vi "Main.vi"() -> ()   [LabVIEW 2022 SP3]
uses:
  MsgTypedef.ctl
  ProcessDataTypedef.ctl
  <vilib>/MakerHub/LINX/Private/Type Defs/LINX Ref.ctl
  <vilib>/MakerHub/LINX/Private/Type Defs/Platform.ctl
  <vilib>/MakerHub/LINX/Private/Type Defs/Interface.ctl
  <vilib>/MakerHub/LINX/Private/Device/Type Defs/LINX Device Config.ctl
  <vilib>/MakerHub/LINX/Private/Device/Type Defs/TCP Config.ctl
  <vilib>/MakerHub/LINX/Private/Device/Type Defs/Channels.ctl
  <vilib>/MakerHub/LINX/Public/Peripherals/Analog/Analog Read 1 Chan.vi
  <vilib>/MakerHub/LINX/Public/Peripherals/Digital/Digital Read 1 Chan.vi
  <vilib>/MakerHub/LINX/Public/Peripherals/Digital/Digital Write 1 Chan.vi
  <vilib>/MakerHub/LINX/Public/Peripherals/Analog/Analog Read N Chans.vi
  <vilib>/MakerHub/LINX/Public/Peripherals/Digital/Digital Read N Chans.vi
  <vilib>/MakerHub/LINX/Public/Peripherals/Digital/Digital Write N Chans.vi
  <vilib>/MakerHub/LINX/Private/Local IO/LinxAnalogRead.vi
  <vilib>/MakerHub/LINX/Public/Utilities/Check Channel.vi
  <vilib>/MakerHub/LINX/Private/Local IO/LinxDigitalRead.vi
  <vilib>/MakerHub/LINX/Private/Local IO/LinxDigitalWrite.vi
  <vilib>/MakerHub/LINX/Public/Utilities/Open Serial.vi
  <vilib>/MakerHub/LINX/Private/Utilties/Generate Error.vi
  <vilib>/MakerHub/LINX/LMH-LINX.lvlib
  <vilib>/MakerHub/LINX/Private/Device/Device.lvlib
panel:
  out "Loop Rate (Hz)":u32
  in  "Close":bool
  in  "Link":bool
  in  "AI Channel":u8
  out "Analog Data":dbl(graph)
  in  "DI Channel":u8=2
  out "DI Value":bool
  in  "DO Value":bool
  in  "DO Channel":u8=13
  in  "Serial Port":refnum<visa-resource-name>
  # "需求....\n1. linx 連結Arduino board \n2. 即時反應IO狀態\n3. 從VI panel 下達IO控制\n4. 可能作狀態觸發 record 記錄到檔案？\n5. 其它想法...."
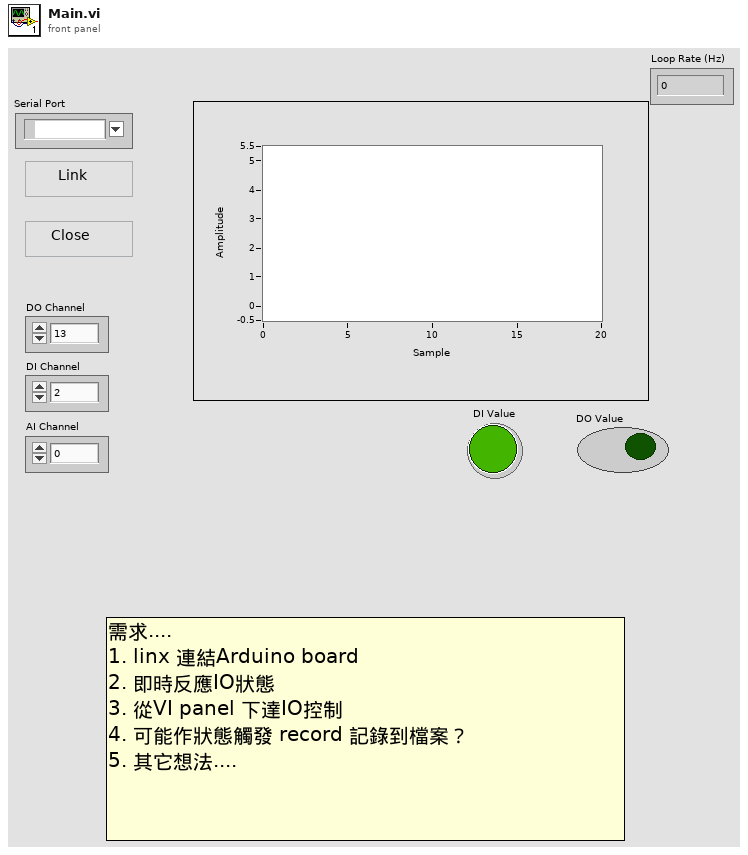
[diagram p1: front panel]
types:
  T1 = typedef "MsgTypedef.ctl" = cluster{"CMD":string, "DATA":variant}
  T2 = typedef "ProcessDataTypedef.ctl" = cluster{"SerialPort":refnum<visa-resource-name>, "DO Channel":u8, "DI Channel":u8, "AI Channel":u8, "AIValue":dbl, "DOStatus":bool, "DIStatus":bool, "DeviceName":string, "LINXResource":T3}
  T3 = typedef "LMH-LINX.lvlib/LINX Ref.ctl" = cluster{"IO":T4, "Interface":T5, "LINX Device Config":T6}
  T4 = typedef "LMH-LINX.lvlib/Platform.ctl" = enum16{"Remote", "Local"}
  T5 = typedef "LMH-LINX.lvlib/Interface.ctl" = enum16{"Serial", "TCP"}
  T6 = typedef "LMH-LINX.lvlib/Device.lvlib/LINX Device Config.ctl" = cluster{"Interface":T5, "COM Port":refnum<visa-resource-name>, "TCP Configuration":T7, "Device Family":u8, "Device ID":u8, "Device Name":string, "TCP Ref":refnum<k5>, "Channels":T8}
  T7 = typedef "LMH-LINX.lvlib/Device.lvlib/TCP Config.ctl" = cluster{"IP Address":string, "Port":u16}
  T8 = typedef "LMH-LINX.lvlib/Channels.ctl" = cluster{"DI":u8[], "DO":u8[], "AI":u8[], "AO":u8[], "PWM":u8[], "QE":u8[], "UART":u8[], "I2C 2":u8[], "SPI":u8[], "CAN":u8[], "Servo":u8[], "AI Ref (V)":dbl, "AI Resolution (Bits)":u8, "AO Ref (V)":dbl, "AO Resolution (Bits)":u8}
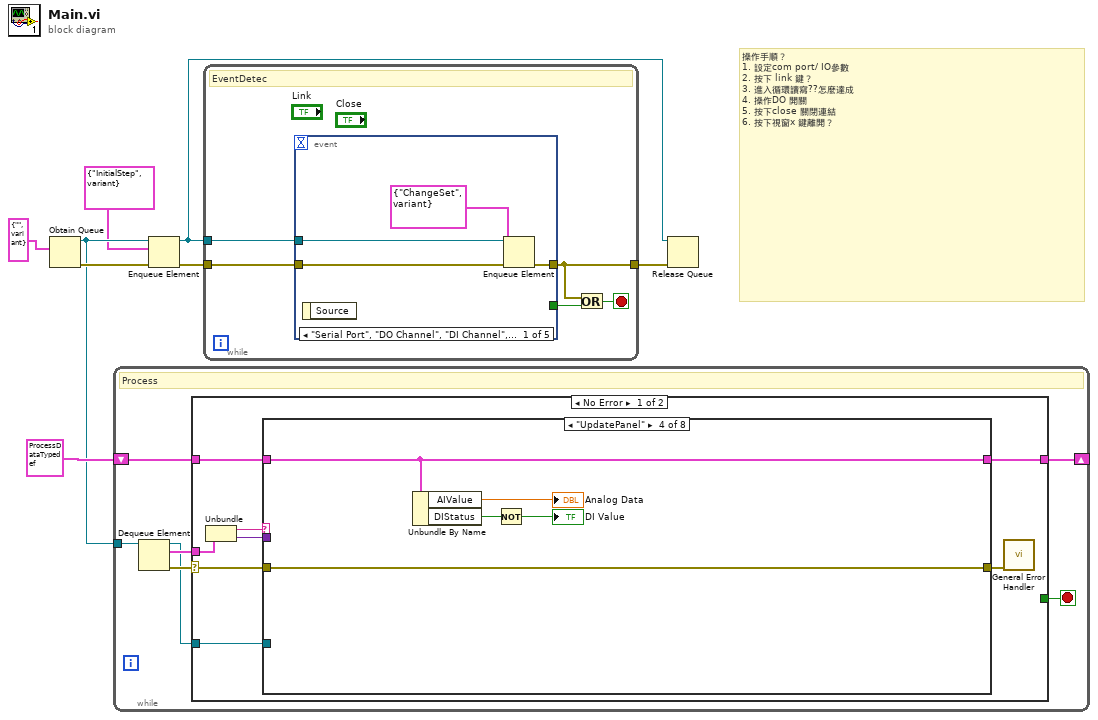
[diagram p0: block diagram]
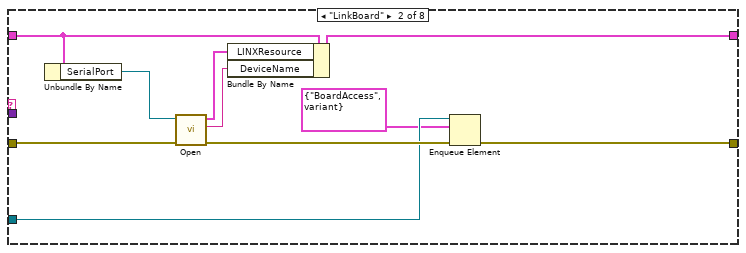
[diagram p3: hidden frame]
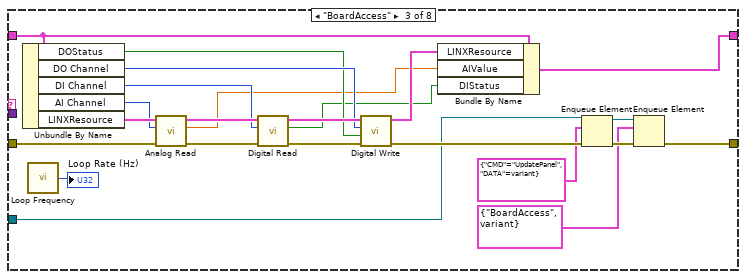
[diagram p4: hidden frame]
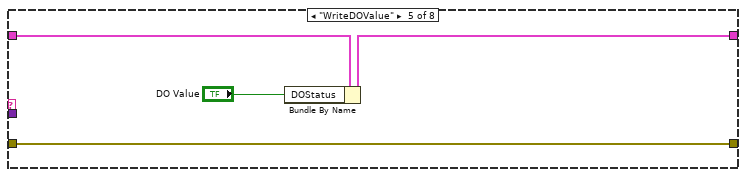
[diagram p5: hidden frame]
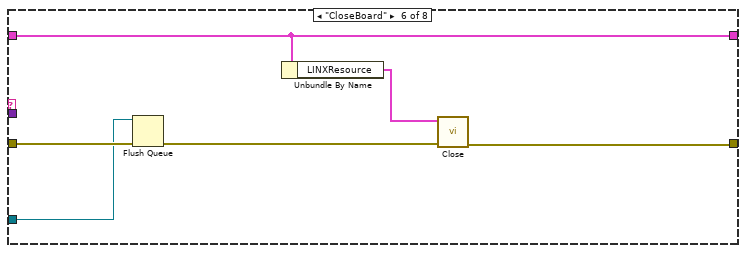
[diagram p6: hidden frame]
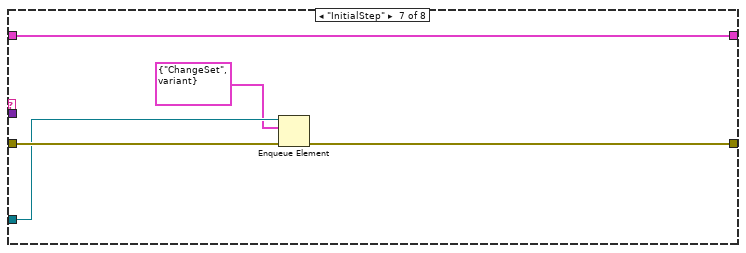
[diagram p7: hidden frame]
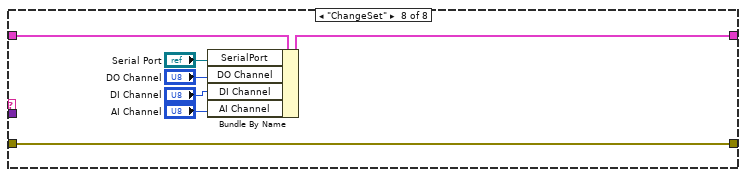
[diagram p8: hidden frame]
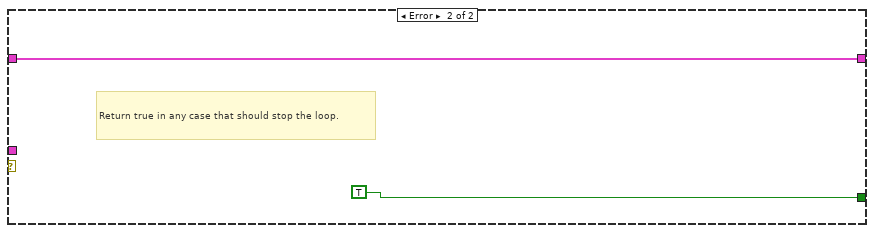
[diagram p9: hidden frame]
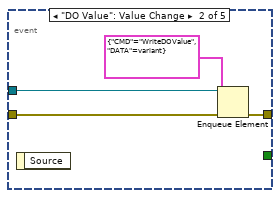
[diagram p10: hidden frame]
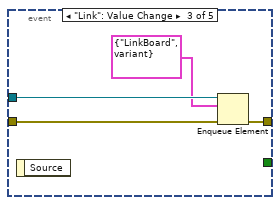
[diagram p11: hidden frame]
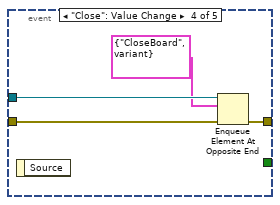
[diagram p12: hidden frame]
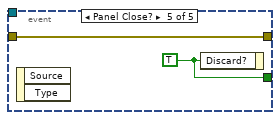
[diagram p13: hidden frame]
diagram:
  # "操作手順？\n1. 設定com port/ IO參數\n2. 按下 link 鍵？\n3. 進入循環讀寫??怎麼達成\n4. 操作DO 開關\n5. 按下close 關閉連結\n6. 按下視窗x 鍵離開？"
  n1 = Obtain Queue(element data type=T1 {"CMD"="", "DATA"=variant}) -> (queue out=w2:refnum<queue>, error out=w8:errorcluster)  [unwired: 4 in, 1 out]
  n2 = while {
    tunnel: w2 -> [w15]
    shift-right: [w11] -> _
    shift-left: T2 {"SerialPort"="", "DO Channel"=13, "DI Channel"=2, "AI Channel"=0, "AIValue"=0.0, "DOStatus"=FALSE, "DIStatus"=FALSE, "DeviceName"="", "LINXResource"={"IO"=enum."Remote", "Interface"=enum."Serial", "LINX Device Config"={"Interface"=enum."Serial", "COM Port"="COM13", "TCP Configuration"={"IP Address"="", "Port"=0}, "Device Family"=1, "Device ID"=1, "Device Name"="myRIO-1900", "TCP Ref"=refnum, "Channels"={"DI"=[0, 1, 2, 3, 4, 5, 6, 7, 8, 9, 10, 11, 12, 13, 14, 15, 16, 17, 18, 19, 20, 21, 22, 23, 24, 25, 26, 27, 28, 29, 30, 31, 32, 33, 34, 35, 36, 37, 38, 39, 40, 41, 42, 43, 44, 45, 46], "DO"=[0, 1, 2, 3, 4, 5, 6, 7, 8, 9, 10, 11, 12, 13, 14, 15, 16, 17, 18, 19, 20, 21, 22, 23, 24, 25, 26, 27, 28, 29, 30, 31, 32, 33, 34, 35, 36, 37, 38, 39, 40, 41, 42, 43, 44, 45, 46], "AI"=[0, 1, 2, 3, 4, 5, 6, 7, 8, 9, 10, 11], "AO"=[], "PWM"=[3, 5, 6, 9, 10], "QE"=[], "UART"=[0, 1], "I2C 2"=[0], "SPI"=[0], "CAN"=[], "Servo"=[], "AI Ref (V)"=0.0, "AI Resolution (Bits)"=0, "AO Ref (V)"=0.0, "AO Resolution (Bits)"=0}}}} -> [w10]
    stop <- w12 stop-if-true
    # "Process"
    n3 = Dequeue Element(queue=w15) -> (queue out=w9:refnum<queue>, element=w13:T1, error out=w14:errorcluster)  [unwired: 2 in, 1 out]
    n4 = case shown="No Error" w14 {
      selector: w14 -> [w21 _]
      tunnel: w13 -> [w23 _]
      tunnel: [_ TRUE] -> w12
      tunnel: [w20 w86] -> w11
      tunnel: w10 -> [w19 w86]
      tunnel: w9 -> [w17 _]
      frame No Error {
        n5 = Unbundle(w23) -> ("CMD"=w22:string, "DATA"=w18:variant)
        n6 = case shown="\"UpdatePanel\"" w22 {
          tunnel: w21 -> [w24 w35 w53 w63 w66 w73 w77 w79]
          tunnel: [w25 w31 w50 w62 w65 w71 w78 w84] -> w20
          tunnel: w19 -> [w25 w33 w52 w62 w67 w71 w78 w85]
          tunnel: w18 -> [_ _ _ _ _ _ _ _]
          tunnel: [w24 w28 w38 w63 w66 w72 w76 w79] -> w16
          tunnel: w17 -> [_ w27 w40 _ _ w68 w75 _]
          frame Default {
          }
          frame "LinkBoard" {
            n7 = Unbundle By Name(w33) -> ("SerialPort"=w32:refnum<visa-resource-name>)
            n8 = call-poly <vilib>:"Open.vi"("Error In"=w35, "Serial Port"=w32) -> ("Error Out"=w34:errorcluster, "Device Name"=w29:string, "LINX Resource"=w30:T3)  [unwired: 7 in]
            n9 = Bundle By Name(cluster=w33, "LINXResource"=w30, "DeviceName"=w29) -> (w31:T2)
            n10 = Enqueue Element(queue=w27, element=T1 {"CMD"="BoardAccess", "DATA"=variant}, error in (no error)=w34) -> (error out=w28:errorcluster)  [unwired: 1 in, 2 out]
          }
          frame "BoardAccess" {
            n11 = Unbundle By Name(w52) -> ("DOStatus"=w45:bool, "DO Channel"=w46:u8, "DI Channel"=w47:u8, "AI Channel"=w48:u8, "LINXResource"=w51:T3)
            n12 = call <vilib>:"Loop Frequency.vi"() -> ("Loop Rate (Hz)"=→"Loop Rate (Hz)":u32)
            n13 = call-poly <vilib>:"Analog Read.vi"("Error In"=w53, "Analog Channel"=w48, "LINX Resource"=w51) -> ("Error Out"=w57:errorcluster, "Voltage"=w44:dbl, "LINX Resource"=w58:T3)  [unwired: 5 in, 1 out]
            n14 = call-poly <vilib>:"Digital Read.vi"("Error In"=w57, "DI Channel"=w47, "LINX Resource"=w58) -> ("Error Out"=w55:errorcluster, "DI Value"=w43:bool, "LINX Resource"=w56:T3)  [unwired: 6 in]
            n15 = call-poly <vilib>:"Digital Write.vi"("Error In"=w55, "Output Value"=w45, "DO Channel"=w46, "LINX Resource"=w56) -> ("Error Out"=w54:errorcluster, "LINX Resource"=w49:T3)  [unwired: 6 in]
            n16 = Bundle By Name(cluster=w52, "LINXResource"=w49, "AIValue"=w44, "DIStatus"=w43) -> (w50:T2)
            n17 = Enqueue Element(queue=w40, element=T1 {"CMD"="UpdatePanel", "DATA"=variant}, error in (no error)=w54) -> (queue out=w37:refnum<queue>, error out=w41:errorcluster)  [unwired: 1 in, 1 out]
            n18 = Enqueue Element(queue=w37, element=T1 {"CMD"="BoardAccess", "DATA"=variant}, error in (no error)=w41) -> (error out=w38:errorcluster)  [unwired: 1 in, 2 out]
          }
          frame "UpdatePanel" {
            n19 = Unbundle By Name(w62) -> ("AIValue"=→"Analog Data":dbl, "DIStatus"=w61:bool)
            n20 = Not(x=w61) -> (.not. x?=→"DI Value":bool)
          }
          frame "WriteDOValue" {
            n21 = Bundle By Name(cluster=w67, "DOStatus"="DO Value") -> (w65:T2)
          }
          frame "CloseBoard" {
            n22 = Flush Queue(queue=w68, error in (no error)=w73) -> (error out=w69:errorcluster)  [unwired: 2 out]
            n23 = Unbundle By Name(w71) -> ("LINXResource"=w70:T3)
            n24 = call <vilib>:"Close.vi"("Error In"=w69, "LINX Resource"=w70) -> ("Error Out"=w72:errorcluster)  [unwired: 9 in]
          }
          frame "InitialStep" {
            n25 = Enqueue Element(queue=w75, element=T1 {"CMD"="ChangeSet", "DATA"=variant}, error in (no error)=w77) -> (error out=w76:errorcluster)  [unwired: 1 in, 2 out]
          }
          frame "ChangeSet" {
            n26 = Bundle By Name(cluster=w85, "SerialPort"="Serial Port", "DO Channel"="DO Channel", "DI Channel"="DI Channel", "AI Channel"="AI Channel") -> (w84:T2)
          }
        }
        n27 = call <vilib>:"General Error Handler.vi"("error in (no error)"=w16) -> ()  [unwired: 10 in, 5 out]
      }
      frame Error {
        # "Return true in any case that should stop the loop."
      }
    }
  }
  n28 = Enqueue Element(queue=w2, element=T1 {"CMD"="InitialStep", "DATA"=variant}, error in (no error)=w8) -> (queue out=w3:refnum<queue>, error out=w4:errorcluster)  [unwired: 1 in, 1 out]
  n29 = while {
    tunnel: w3 -> [w92]
    tunnel: w4 -> [w91]
    tunnel: [w88] -> w7
    stop <- w89 stop-if-true
    # "EventDetec"
    n30 = event shown="[0] \"Serial Port\", \"DO Channel\", \"DI Channel\", \"AI Channel\": Value Change" {
      selector: _ -> [_ _ _ _ _]
      dyn-events: _ -> [_ _ _ _ _]
      timeout: _ -> [_ _ _ _ _]
      tunnel: w92 -> [w96 w100 w104 w108 _]
      tunnel: w91 -> [w95 w99 w103 w107 w110]
      tunnel: [w94 w98 w102 w106 w110] -> w88
      tunnel: [_ _ _ _ w109] -> w90
      event "Serial Port", "DO Channel", "DI Channel", "AI Channel": Value Change {
        n31 = event-data() -> ()  [unwired: 1 in, 1 out]
        n32 = Enqueue Element(queue=w96, element=T1 {"CMD"="ChangeSet", "DATA"=variant}, error in (no error)=w95) -> (error out=w94:errorcluster)  [unwired: 1 in, 2 out]
      }
      event "DO Value": Value Change {
        n33 = event-data() -> ()  [unwired: 1 in, 1 out]
        n34 = Enqueue Element(queue=w100, element=T1 {"CMD"="WriteDOValue", "DATA"=variant}, error in (no error)=w99) -> (error out=w98:errorcluster)  [unwired: 1 in, 2 out]
      }
      event "Link": Value Change {
        n35 = event-data() -> ()  [unwired: 1 in, 1 out]
        n36 = Enqueue Element(queue=w104, element=T1 {"CMD"="LinkBoard", "DATA"=variant}, error in (no error)=w103) -> (error out=w102:errorcluster)  [unwired: 1 in, 2 out]
      }
      event "Close": Value Change {
        n37 = event-data() -> ()  [unwired: 1 in, 1 out]
        n38 = Enqueue Element At Opposite End(queue=w108, element=T1 {"CMD"="CloseBoard", "DATA"=variant}, error in (no error)=w107) -> (error out=w106:errorcluster)  [unwired: 1 in, 2 out]
      }
      event Panel Close? {
        w109 = TRUE ("Discard?")
        n39 = event-data() -> ()  [unwired: 1 in, 2 out]
        n40 = event-data("Discard?"=w109) -> ()  [unwired: 1 in, 1 out]
      }
    }
    n41 = Or(x=w88, y=w90) -> (x .or. y?=w89:bool)
  }
  n42 = Release Queue(queue=w3, error in (no error)=w7) -> ()  [unwired: 1 in, 3 out]
